vi "Change GFG Boolean Control Property.vi"(7 "Change GFG Boolean Control Property_Command":T1, 8 "error in (no error)":errorcluster, 11 "GFG Boolean Control name IN (.CtrlRef)":string) -> (0 "error out":errorcluster)   [LabVIEW 2012]
doc: "SciScan 1.2 160622"
uses:
  Change GFG Boolean Control Property_Command.ctl
  GFG/GFG library.lvlib
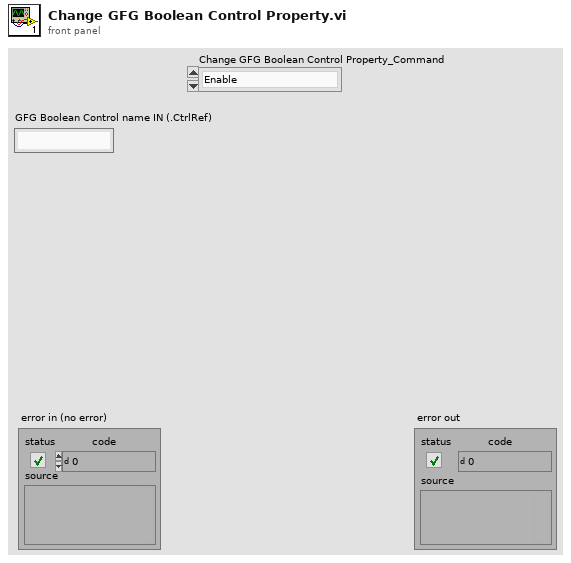
[diagram p1: front panel]
types:
  T1 = typedef "Change GFG Boolean Control Property_Command.ctl" = enum16{"Enable", "Disable", "Disable and Grey", "Start Blinking", "Stop Blinking"}
  T2 = enum8{"Enabled", "Disabled", "Disabled and Grayed Out"}
  T3 = cluster{"WaveformChartRef":refnum<vi>, "DigitalRef":refnum<vi>, "ArrayRef":refnum<vi>, "TabControlRef":refnum<vi>, "EnumRef":refnum<vi>, "RingRef":refnum<vi>, "BooleanRef":refnum<vi>, "KnobRef":refnum<vi>, "SlideRef":refnum<vi>, "PathRef":refnum<vi>, "StringRef":refnum<vi>, "ComboBox":refnum<vi>, "WaveformGraphRef":refnum<vi>}
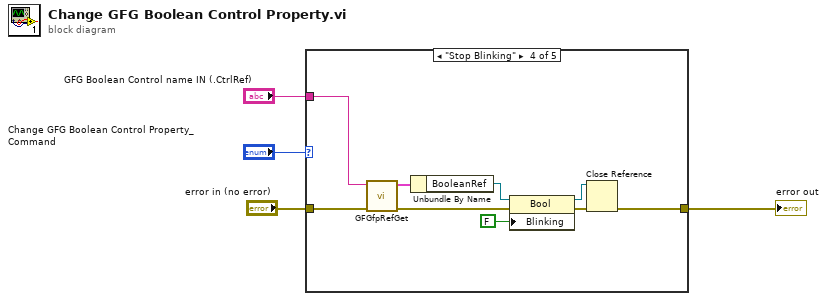
[diagram p0: block diagram]
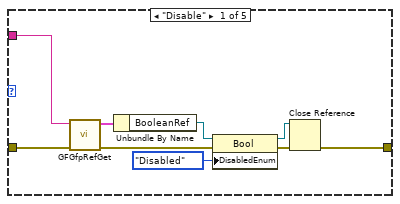
[diagram p2: hidden frame]
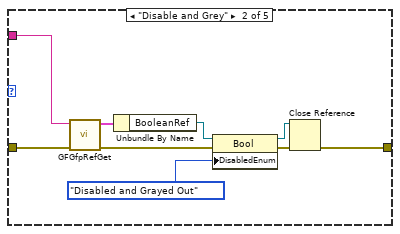
[diagram p3: hidden frame]
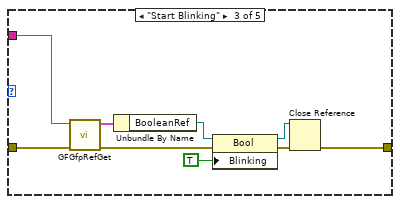
[diagram p4: hidden frame]
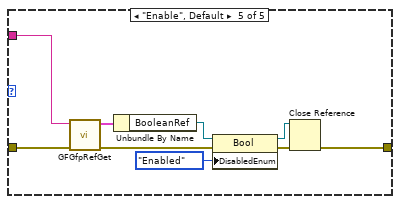
[diagram p5: hidden frame]
diagram:
  n1 = case shown="\"Stop Blinking\"" "Change GFG Boolean Control Property_Command" {
    tunnel: "error in (no error)" -> [w8 w17 w26 w35 w44]
    tunnel: "GFG Boolean Control name IN (.CtrlRef)" -> [w7 w16 w25 w34 w43]
    tunnel: [w6 w15 w24 w33 w42] -> w1
    frame "Disable" {
      n2 = call "GFGfpRefGet.vi"("error in (no error)"=w8, "Variable Name in"=w7) -> ("error out"=w11:errorcluster, "output cluster"=w13:T3)  [unwired: 8 in]
      n3 = Unbundle By Name(w13) -> ("BooleanRef"=w12:refnum<vi>)
      n4 = property class="Bool"(reference=w12, error in=w11, "DisabledEnum"=T2."Disabled" ("Disabled")) -> (reference out=w9:refnum<vi>, error out=w10:errorcluster)
      n5 = Close Reference(reference=w9, error in (no error)=w10) -> (error out=w6:errorcluster)
    }
    frame "Disable and Grey" {
      n6 = call "GFGfpRefGet.vi"("error in (no error)"=w17, "Variable Name in"=w16) -> ("error out"=w20:errorcluster, "output cluster"=w22:T3)  [unwired: 8 in]
      n7 = Unbundle By Name(w22) -> ("BooleanRef"=w21:refnum<vi>)
      n8 = property class="Bool"(reference=w21, error in=w20, "DisabledEnum"=T2."Disabled and Grayed Out" ("Disabled")) -> (reference out=w18:refnum<vi>, error out=w19:errorcluster)
      n9 = Close Reference(reference=w18, error in (no error)=w19) -> (error out=w15:errorcluster)
    }
    frame "Start Blinking" {
      n10 = call "GFGfpRefGet.vi"("error in (no error)"=w26, "Variable Name in"=w25) -> ("error out"=w29:errorcluster, "output cluster"=w31:T3)  [unwired: 8 in]
      n11 = Unbundle By Name(w31) -> ("BooleanRef"=w30:refnum<vi>)
      n12 = property class="Bool"(reference=w30, error in=w29, "Blinking"=TRUE) -> (reference out=w27:refnum<vi>, error out=w28:errorcluster)
      n13 = Close Reference(reference=w27, error in (no error)=w28) -> (error out=w24:errorcluster)
    }
    frame "Stop Blinking" {
      n14 = call "GFGfpRefGet.vi"("error in (no error)"=w35, "Variable Name in"=w34) -> ("error out"=w38:errorcluster, "output cluster"=w40:T3)  [unwired: 8 in]
      n15 = Unbundle By Name(w40) -> ("BooleanRef"=w39:refnum<vi>)
      n16 = property class="Bool"(reference=w39, error in=w38, "Blinking"=FALSE) -> (reference out=w36:refnum<vi>, error out=w37:errorcluster)
      n17 = Close Reference(reference=w36, error in (no error)=w37) -> (error out=w33:errorcluster)
    }
    frame "Enable", Default {
      n18 = call "GFGfpRefGet.vi"("error in (no error)"=w44, "Variable Name in"=w43) -> ("error out"=w47:errorcluster, "output cluster"=w49:T3)  [unwired: 8 in]
      n19 = Unbundle By Name(w49) -> ("BooleanRef"=w48:refnum<vi>)
      n20 = property class="Bool"(reference=w48, error in=w47, "DisabledEnum"=T2."Enabled" ("Disabled")) -> (reference out=w45:refnum<vi>, error out=w46:errorcluster)
      n21 = Close Reference(reference=w45, error in (no error)=w46) -> (error out=w42:errorcluster)
    }
  }
  "error out" <- w1
